vi "Execute Callback.vi"(8 "Write Status":errorcluster, 11 "IWriteExecutionPolicy in":refnum<class "IWriteExecutionCallback.lvclass">) -> ()   [LabVIEW 2019, in "MessagingInterfaces.lvlib" / "IWriteExecutionCallback.lvclass"]
uses:
  <vilib>/gpm_packages/@cs/Network-interface/Source/MessagingInterfaces/IWriteExecutionCallback/IWriteExecutionCallback.lvclass
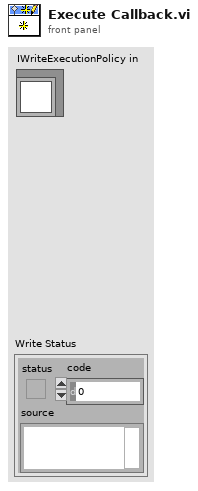
[diagram p1: front panel]
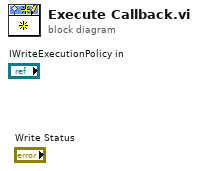
[diagram p0: block diagram]
diagram:
